vi "Module Pong.vi"(8 "error in":errorcluster) -> (0 "error out":errorcluster)   [LabVIEW 2015, in "Generic Module Library.lvlib" / "Template G_Module.lvlib"]
uses:
  Template G_Module.lvlib
  Private Controls/Event Item.ctl
  Broadcast Support/Broadcast Actions.ctl
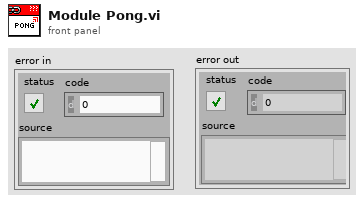
[diagram p1: front panel]
types:
  T1 = typedef "Generic Module Library.lvlib/Template G_Module.lvlib/Broadcast Actions.ctl" = enum16{"Create", "Get", "Destroy"}
  T2 = typedef "Generic Module Library.lvlib/Template G_Module.lvlib/Event Item.ctl" = cluster{"Event Data":variant}
  T3 = typedef "Generic Module Library.lvlib/Template G_Module.lvlib/Broadcast List.ctl" = cluster{"Module Started":refnum<user-event>, "Module Error":refnum<user-event>, "Module Pong":refnum<user-event>, "Module Status":refnum<user-event>, "Module Stopping":refnum<user-event>, "Module Stopped":refnum<user-event>, "Module Reinitialized":refnum<user-event>}
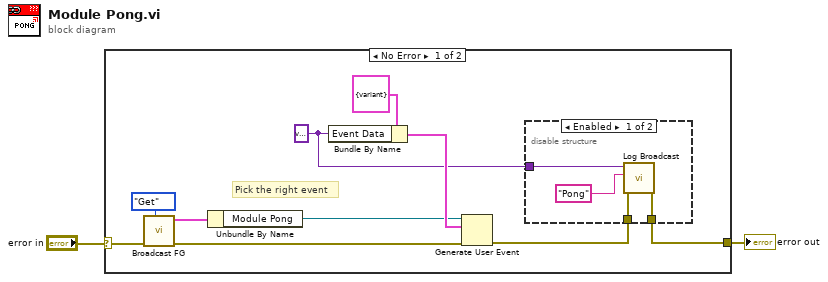
[diagram p0: block diagram]
diagram:
  n1 = case shown="No Error" "error in" {
    selector: "error in" -> [w6 w18]
    tunnel: [w4 w18] -> w2
    frame No Error {
      w3 = variant ("Broadcast Data")
      # "Pick the right event"
      n2 = call "Broadcast FG.vi"("Broadcast Actions"=Broadcast_Actions."Get", "error in"=w6) -> ("error out"=w12:errorcluster, "Broadcast List"=w8:T3)  [unwired: 8 in]
      n3 = Unbundle By Name(w8) -> ("Module Pong"=w7:refnum<user-event>)
      n4 = Bundle By Name(cluster=T2 {"Event Data"=variant} ("Broadcast Item"), "Event Data"=w3) -> (w10:T2)
      n5 = Generate User Event(user event=w7, event data cluster=w10, error in=w12) -> (error out=w5:errorcluster)  [unwired: 1 in, 1 out]
      n6 = disable-structure shown="Enabled" {
        disable-tunnel: w5 -> [w16 w17]
        disable-tunnel: [w15 w17] -> w4
        disable-tunnel: w3 -> [w13 _]
        frame Enabled {
          n7 = call "Log Broadcast.vi"("error in"=w16, "Broadcast Name"="Pong", "Message Data In"=w13) -> ("error out"=w15:errorcluster)  [unwired: 8 in]
        }
        frame Disabled {
        }
      }
    }
    frame Error {
    }
  }
  "error out" <- w2
